vi "Keyence_VS150.vi"(9 "Setting Value":string, 10 "Row No.":string, 11 "Coulumn No.":string) -> (3 "Inspection_Result":bool)   [LabVIEW 2024, in "Keyence_VS150.lvlib"]
doc: "This template is for the Queued Message Handler design pattern.\n\nThe Event Handling Loop generates messages based on user interface actions.\n\nThe Message Handling Loop processes messages generated by the Event Handling Loop, or by other messages. The messages are string values, so new messages can be added easily to the Message Cases case structure in the Message Handling Loop. Each message cluster can also provide an optional value for Message Data, which is a variant that can be converted to whatever message-specific data is required."
uses:
  Keyence_VS150.lvlib
  controls/UI Data.ctl
  Settings/support/Camera.ctl
  <userlib>/_OpenG.lib/array/array.llb/Search 1D Array (String)__ogtk.vi
  <vilib>/Utility/error.llb/Error Cluster From Error Code.vi
  <vilib>/ErrorRing/Error Ring.xnode
  Keysight_34461a/support/Message Queue/Message Queue.lvlib
  support/User Event - Stop/User Event - Stop.lvlib
  support/Message Queue/Message Queue.lvlib
  <userlib>/_OpenG.lib/string/string.llb/openg_string.lvlib
  Launcher/Launcher_DTU.lvlib
  <userlib>/_OpenG.lib/array/array.llb/openg_array.lvlib
  Settings/Setting_Screen.lvlib
panel:
  out "Gray Intensity Value":string
  in  "Row No. 2":string
  in  "Coulumn No. 2":string
  in  "Setting Value 2":string
  in  "Storage 2":string
  in  "Program No 2":string
  out "data 2":string
  out "Get Mode 2":string
  in  "Change_Program":bool
  out "RX/RY":string
  out "RX,RY":string
  out "status":bool
  in  "Trigger":bool
  in  "Total_Result":T1
  out "DTU 2":string[][](array[string])
  out "DTU1":string[][](array[string])
  out "DTU_Failed_Inspections_Array":string[](array[string])
  out "Fail":i32[](array[numeric])
  out "Inspection_names":string[](array[string])
  out "Result_Values":string[](array[string])
  out "DTU_Failed_Inspections":string
  in  "Config":string
  out "queue name 2":string
  out "queue name":string
  in  "ip address":string="169.254.73.187"
  in  "DUT":string
  out "Result Value":string[](array[string])
  out "Array of Strings":string[](array[string])
  out "data out":string
  out "data":string
  out "Get Mode":string
  in  "Program No":string
  in  "Storage":string
  out "Display <Replace Me>":string
  in  "Exit":bool
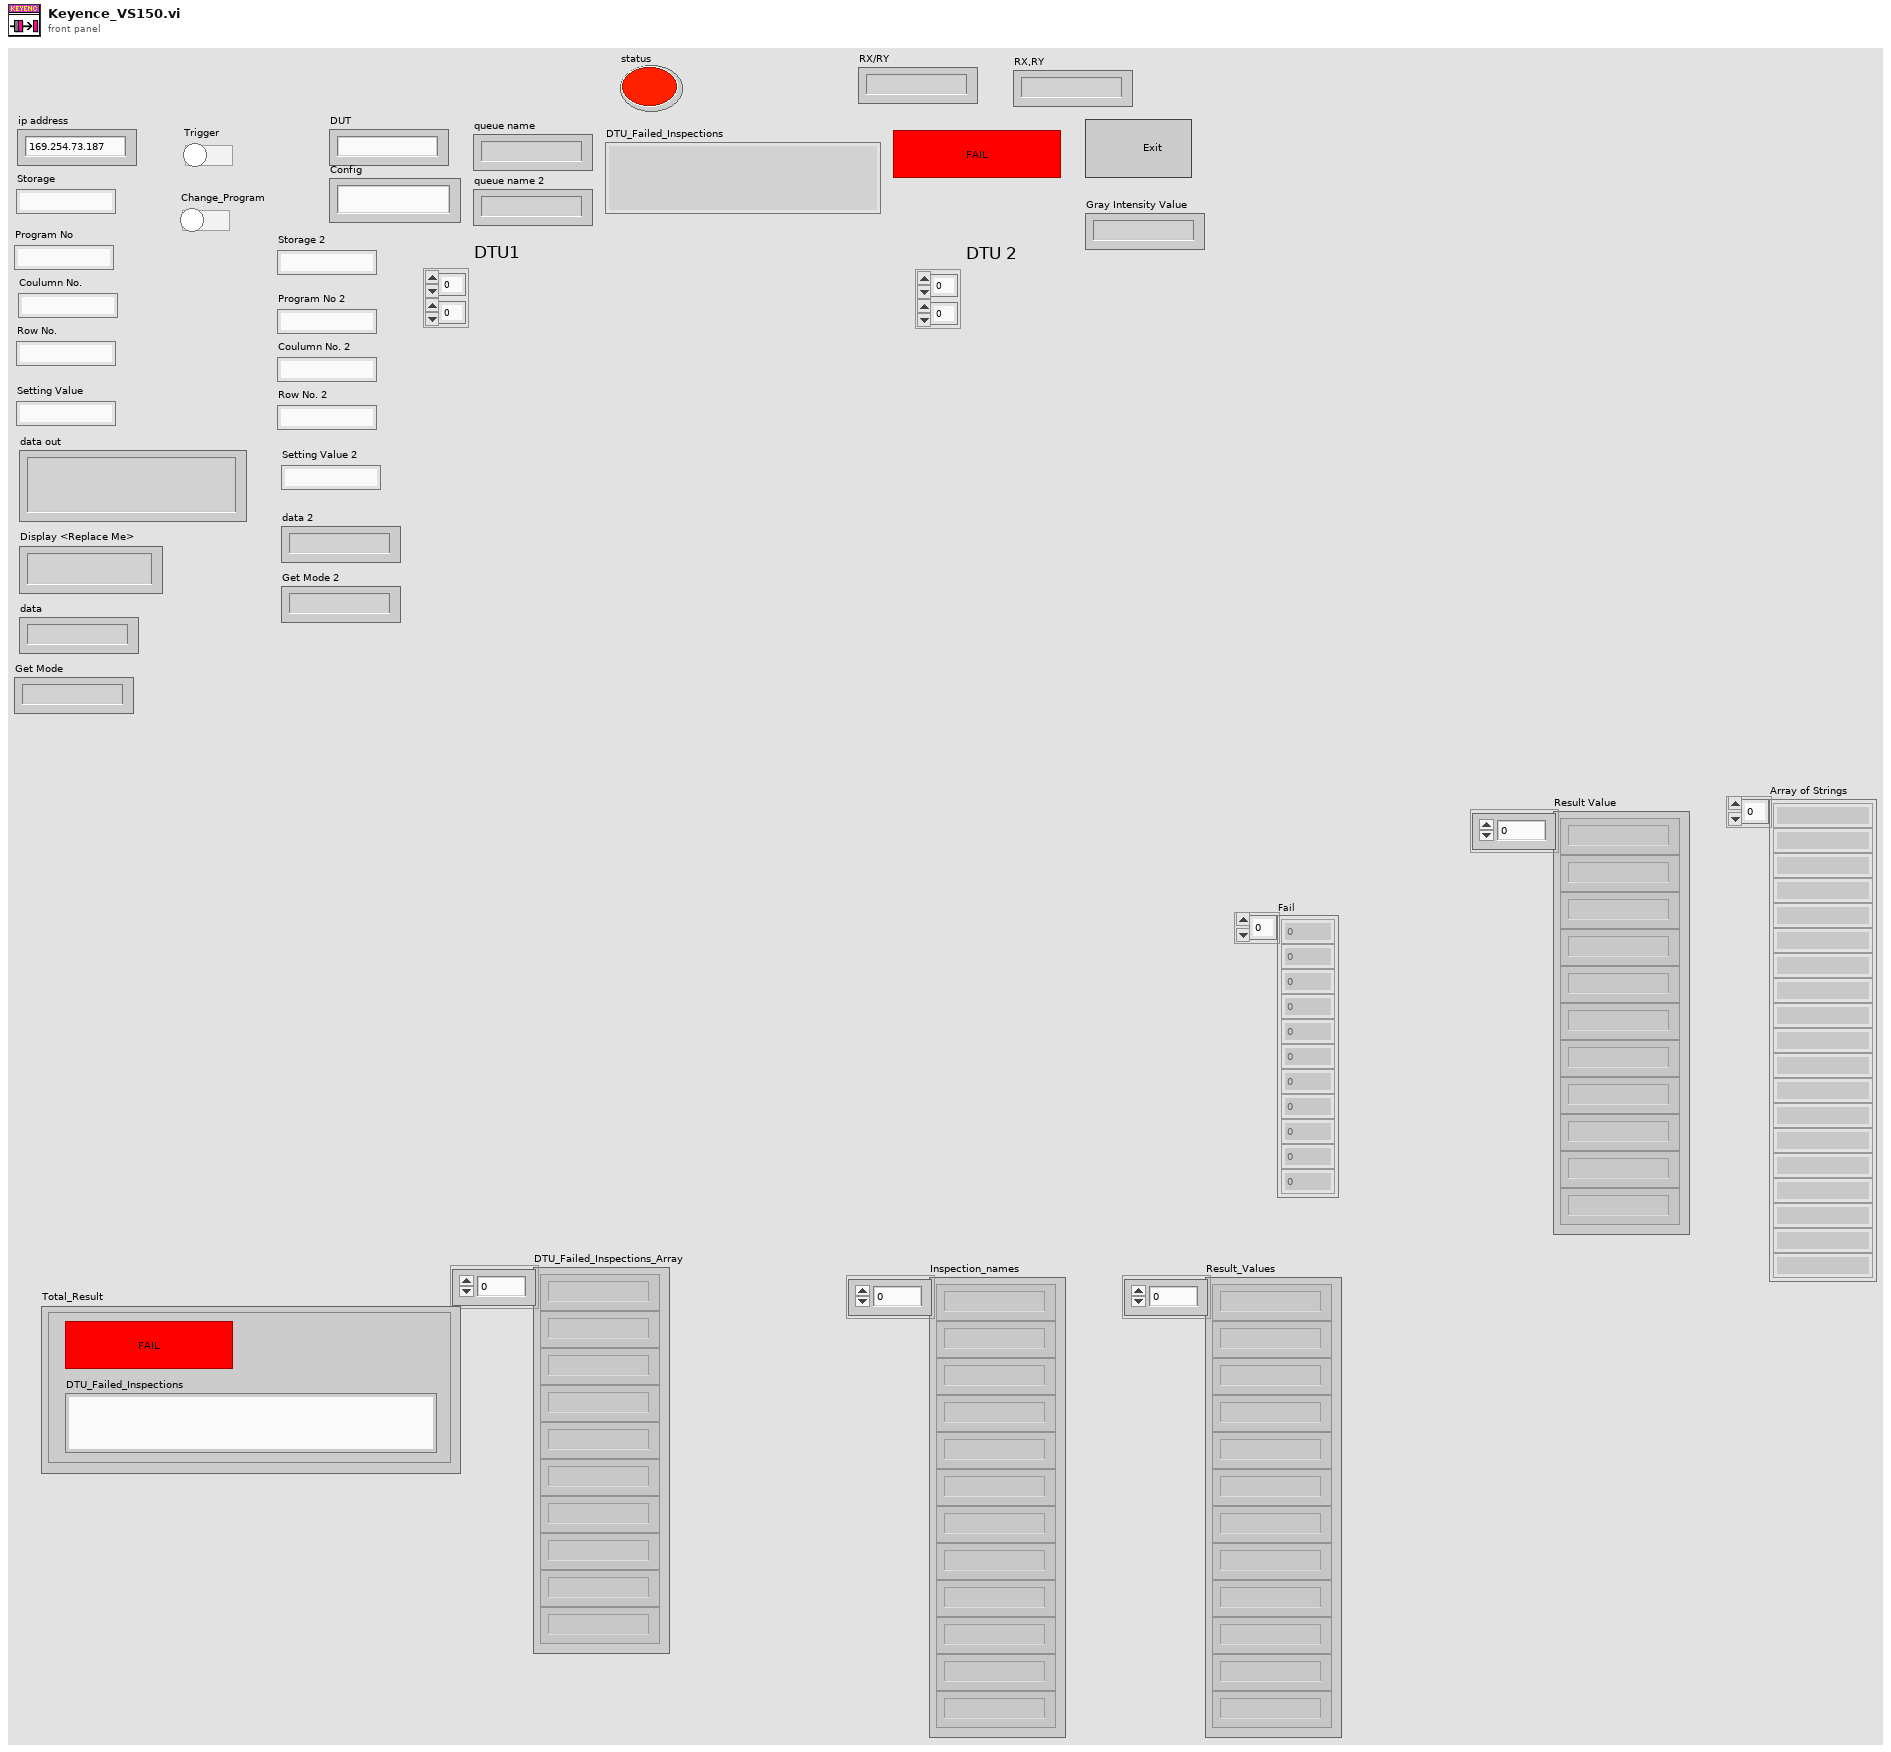
[diagram p1: front panel]
types:
  T1 = cluster{"Inspection_Result 2":bool, "DTU_Failed_Inspections":string}
  T2 = typedef "Keyence_VS150.lvlib/UI Data.ctl" = cluster{"Boolean <Replace Me>":bool, "String <Replace Me>":string, "Numeric <Replace Me>":dbl, "Data Display Ref":refnum<vi>, "Exit Button Ref":refnum<vi>, "connection ID":refnum<k5>, "data out":string, "notifier out":refnum<notifier>, "DUT":string, "Config":string, "Keyence_VS150":refnum<queue>, "Result Value":string[], "Inspection_Result":bool, "Total_Result":cluster{"Inspection_Result 2":bool, "DTU_Failed_Inspections":string}, "Camera":T3, "Camera_Program No":string, "DUT1":string, "DUT2":string}
  T3 = typedef "Setting_Screen.lvlib/Camera.ctl" = cluster{"Trigger":bool, "Prog No.":string, "Delay":bool, "Delay time":dbl, "Storage":string, "Col no.":string, "Row no.":string}
  T4 = typedef "Keyence_VS150.lvlib/Message Queue.lvlib/All Message Queues.ctl" = cluster{"UI":refnum<queue>, "QSM":refnum<queue>}
  T5 = cluster{"Message":string, "Message Data":variant}
  T6 = enum16{"Read", "Write", "All_sections", "All_values", "Remove key&section"}
  T7 = cluster{"Status":string, "Free/inuse":bool, "Action":string}
  T8 = enum16{"Standard", "Buffered", "CRLF", "Immediate"}
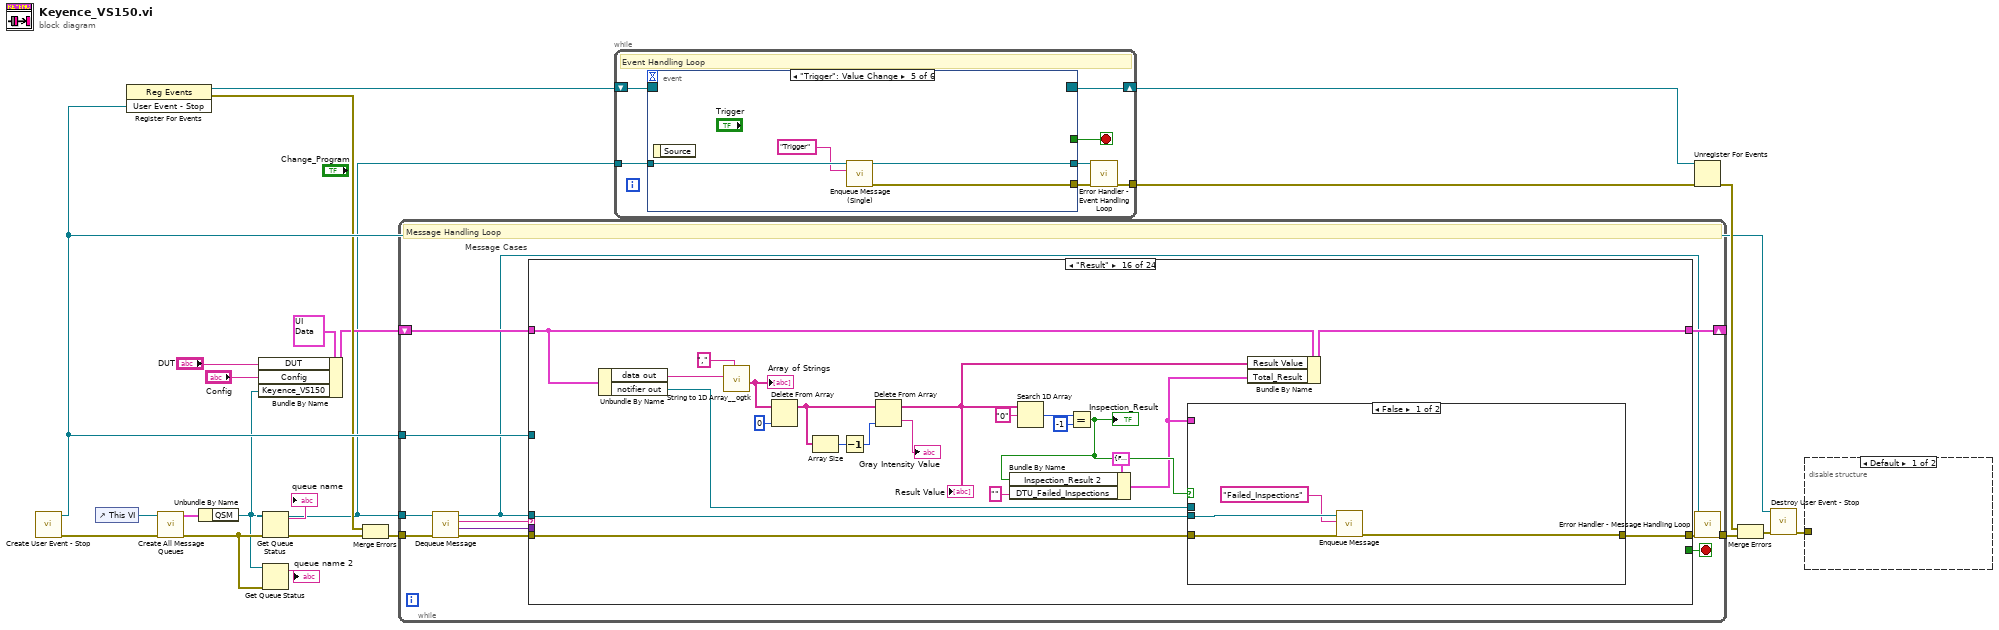
[diagram p0: block diagram]
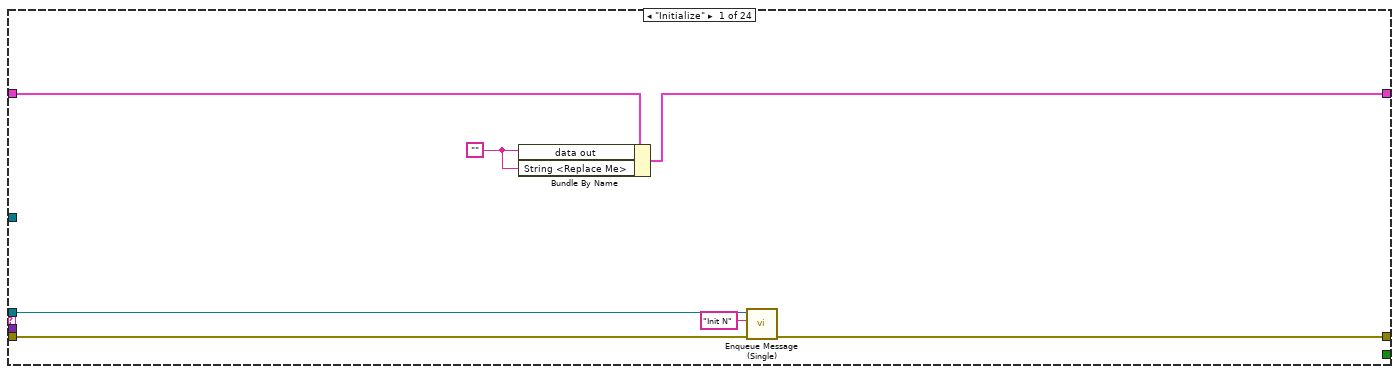
[diagram p2: hidden frame]
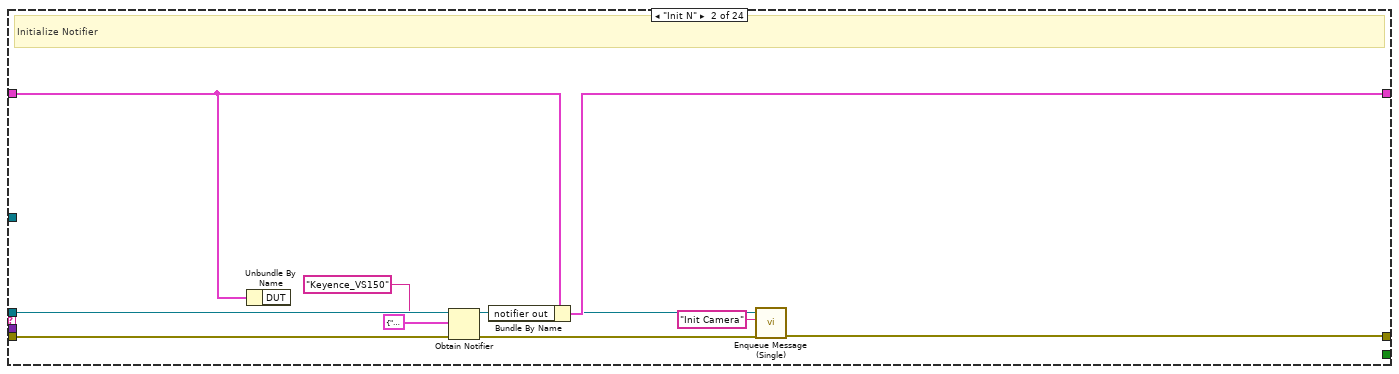
[diagram p3: hidden frame]
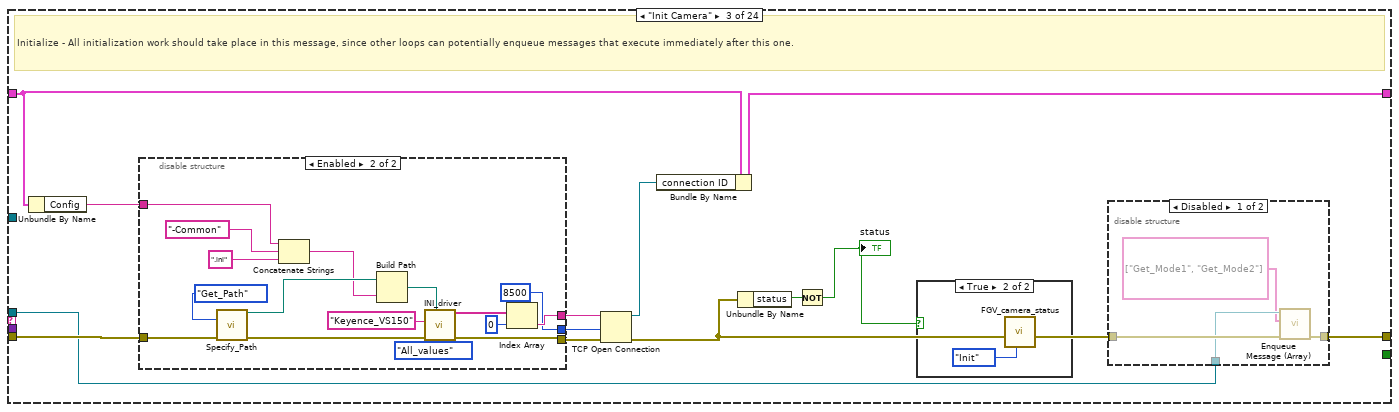
[diagram p4: hidden frame]
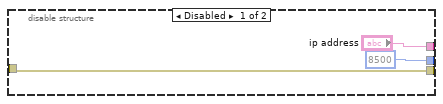
[diagram p7: hidden frame]
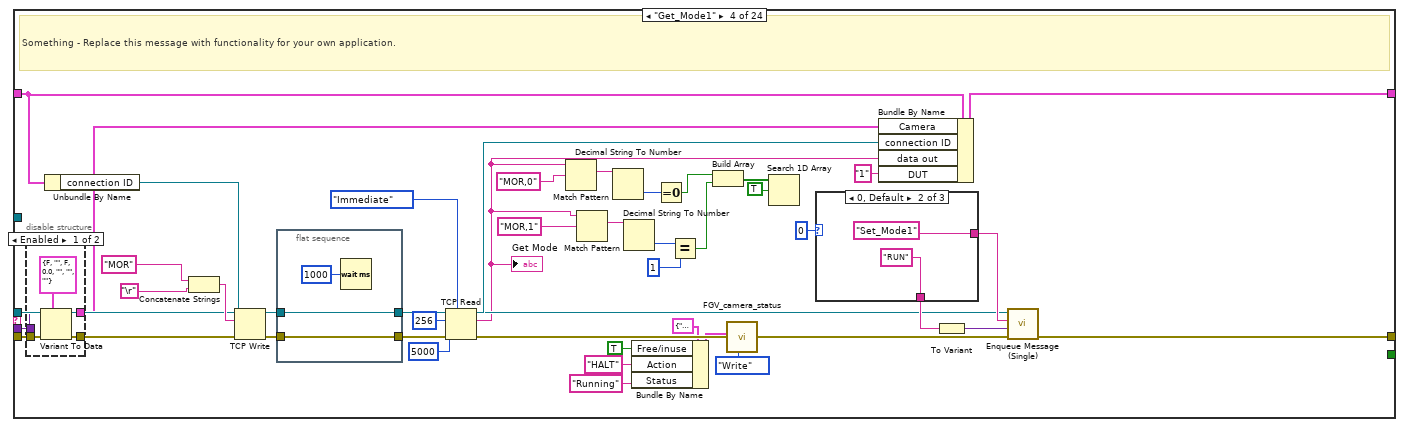
[diagram p8: hidden frame]
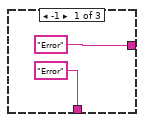
[diagram p10: hidden frame]
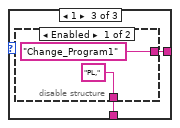
[diagram p11: hidden frame]
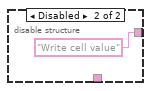
[diagram p12: hidden frame]
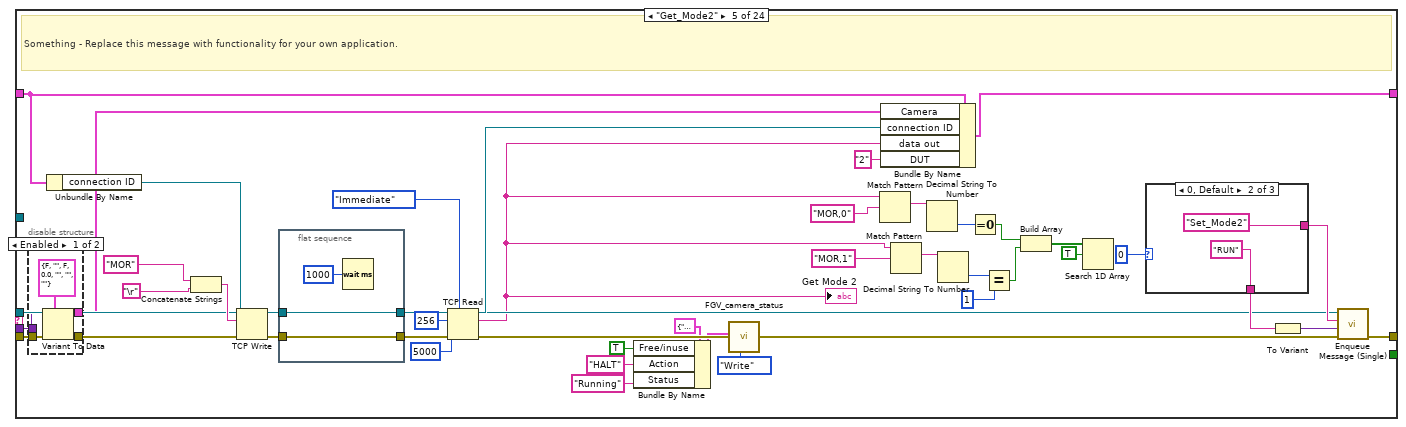
[diagram p13: hidden frame]
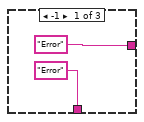
[diagram p15: hidden frame]
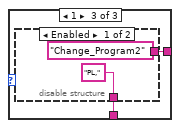
[diagram p16: hidden frame]
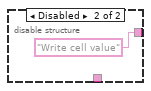
[diagram p17: hidden frame]
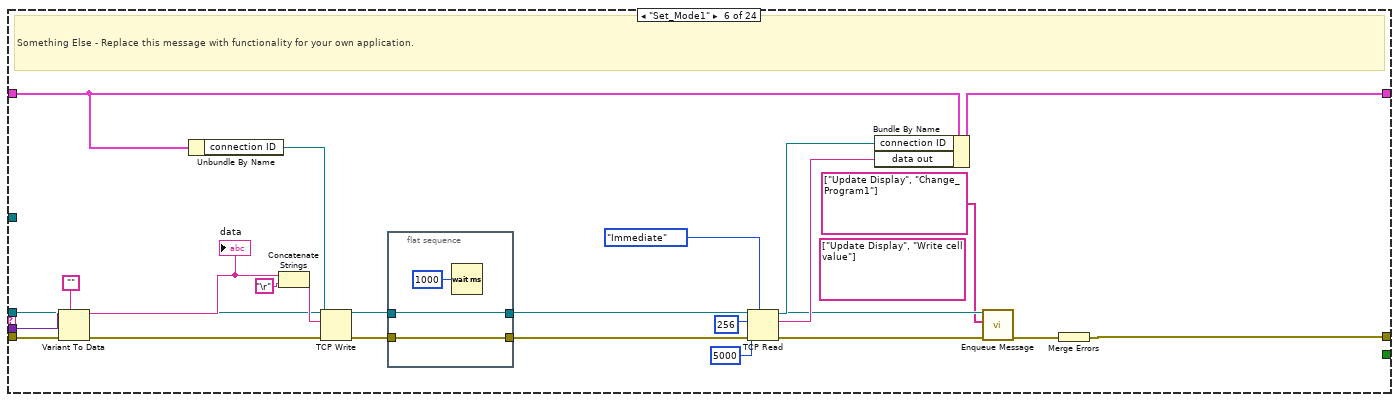
[diagram p18: hidden frame]
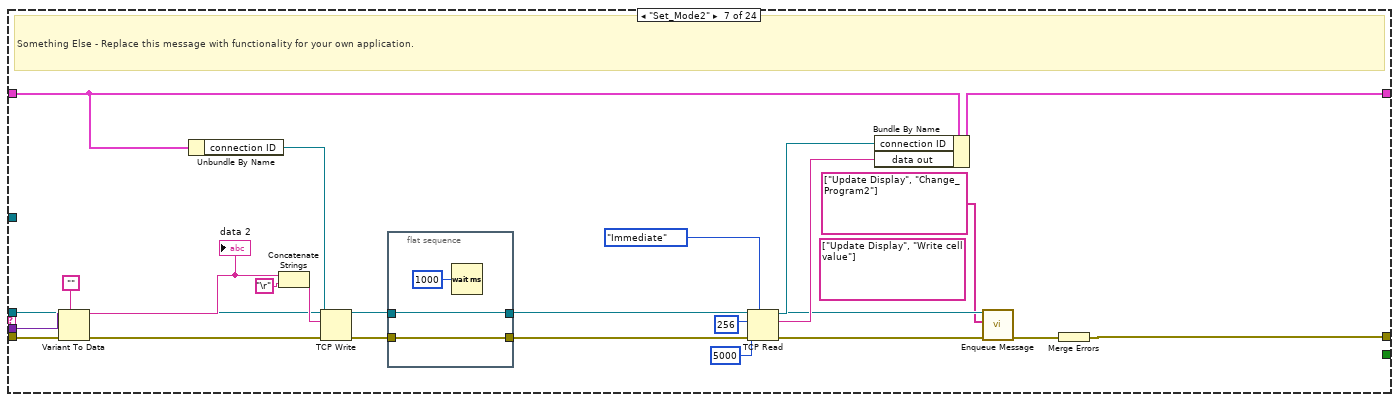
[diagram p19: hidden frame]
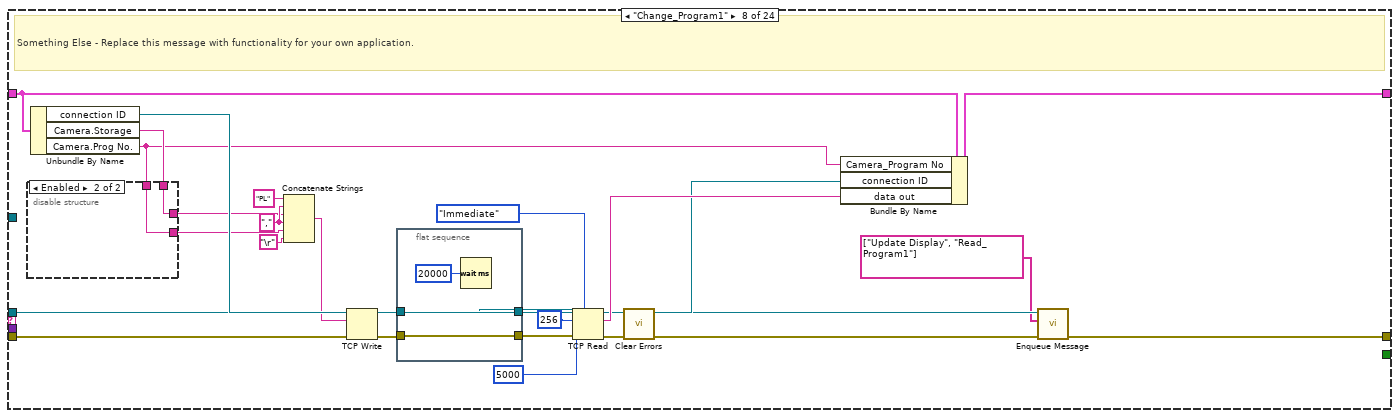
[diagram p20: hidden frame]
diagram:
  n1 = call "Create User Event - Stop.vi"() -> ("error out"=w21:errorcluster, "User Event - Stop"=w14:refnum<user-event>)  [unwired: 10 in]
  n2 = control-ref of="This VI"() -> (w9:refnum<vi>)
  n3 = register-events(w14) -> (reference out=w15:refnum<event-registration>, error out=w12:errorcluster)  [unwired: 2 in]
  n4 = call "Create All Message Queues.vi"("error in (no error)"=w21, "This VI"=w9) -> ("error out"=w3:errorcluster, "Message Queues out"=w23:T4)  [unwired: 8 in]
  n5 = Unbundle By Name(w23) -> ("QSM"=w1:refnum<queue>)
  n6 = Bundle By Name(cluster=T2 {"Boolean <Replace Me>"=FALSE, "String <Replace Me>"="", "Numeric <Replace Me>"=0.0, "Data Display Ref"=refnum, "Exit Button Ref"=refnum, "connection ID"=refnum, "data out"="", "notifier out"=refnum, "DUT"="", "Config"="", "Keyence_VS150"=refnum, "Result Value"=[], "Inspection_Result"=FALSE, "Total_Result"={"Inspection_Result 2"=FALSE, "DTU_Failed_Inspections"=""}, "Camera"={"Trigger"=FALSE, "Prog No."="", "Delay"=FALSE, "Delay time"=0.0, "Storage"="", "Col no."="", "Row no."=""}, "Camera_Program No"="", "DUT1"="", "DUT2"=""} ("Data Cluster"), "DUT"="DUT", "Config"="Config", "Keyence_VS150"=w1) -> (w10:T2)
  n7 = Get Queue Status(queue=w1, error in (no error)=w3) -> (queue out=w5:refnum<queue>, queue name=→"queue name":string, error out=w4:errorcluster)  [unwired: 1 in, 5 out]
  n8 = Get Queue Status(queue=w1, error in (no error)=w3) -> (queue name=→"queue name 2":string)  [unwired: 1 in, 7 out]
  n9 = Merge Errors(w12, w4) -> (w13:errorcluster)
  n10 = while {
    tunnel: w5 -> [w27]
    shift-right: [w34] -> _
    shift-left: w10 -> [w35]
    tunnel: w14 -> [w32]
    tunnel: w13 -> [w31]
    tunnel: [w25] -> w22
    stop <- w33 stop-if-true
    # "Message Handling Loop"
    n11 = call "Dequeue Message.vi"("error in (no error)"=w31, "Message Queue"=w27) -> ("error out"=w30:errorcluster, "Message Data"=w28:variant, "Message"=w29:string, "dup Message Queue"=w26:refnum<queue>)  [unwired: 6 in]
    n12 = case "Message Cases" shown="\"Result\"" w29 {
      selector: w29 -> [_ _ _ _ _ _ _ _ _ _ _ _ _ _ _ _ _ _ _ _ _ _ _ w780]
      tunnel: w26 -> [w37 w45 w54 w115 w176 w218 w245 w283 w316 w337 w384 w451 w502 w546 w574 w604 _ _ _ _ _ w763 w779 _]
      tunnel: w30 -> [w39 w51 w60 w130 w191 w228 w255 w284 w317 w338 w385 w445 w496 w539 w567 w607 w645 w712 w740 w750 w755 w758 w771 _]
      tunnel: [w38 w47 w53 w101 w162 w235 w262 w291 w324 w343 w390 w452 w503 w548 w556 w606 w653 w711 w741 w744 w753 w764 w776 w781] -> w24
      tunnel: w35 -> [w42 w44 w59 w122 w183 w222 w249 w288 w321 w334 w381 w442 w493 w536 w565 w609 w652 w715 w739 w749 w754 w756 w770 w782]
      tunnel: [w40 w49 w64 w121 w182 w221 w248 w287 w320 w340 w387 w441 w492 w535 w564 w608 w652 w715 w739 w749 w754 w756 w770 w782] -> w34
      tunnel: [_ _ _ _ _ _ _ _ _ _ _ _ _ _ _ _ _ _ _ _ _ _ TRUE _] -> w33
      tunnel: w28 -> [_ _ _ w99 w160 w225 w252 _ _ _ _ _ _ _ _ _ _ _ _ w748 _ _ w772 _]
      tunnel: w32 -> [_ _ _ _ _ _ _ _ _ _ _ _ _ _ _ _ _ _ _ _ _ _ w775 _]
      frame "Initialize" {
        w41 = "" ("data out")
        n13 = Bundle By Name(cluster=w42, "data out"=w41, "String <Replace Me>"=w41) -> (w40:T2)
        n14 = call "Enqueue Message (Single).vi"("error in (no error)"=w39, "Message"="Init N", "Message Queue"=w37) -> ("error out"=w38:errorcluster)  [unwired: 7 in, 1 out]
      }
      frame "Init N" {
        # "Initialize Notifier"
        n15 = Unbundle By Name(w44) -> ()  [unwired: 1 out]
        n16 = Obtain Notifier(name (unnamed)="Keyence_VS150", notification data type=T5 {"Message"="", "Message Data"=variant} ("notification"), error in (no error)=w51) -> (notifier out=w50:refnum<notifier>, error out=w48:errorcluster)  [unwired: 1 in, 1 out]
        n17 = Bundle By Name(cluster=w44, "notifier out"=w50) -> (w49:T2)
        n18 = call "Enqueue Message (Single).vi"("error in (no error)"=w48, "Message"="Init Camera", "Message Queue"=w45) -> ("error out"=w47:errorcluster)  [unwired: 7 in, 1 out]
      }
      frame "Init Camera" {
        # "Initialize - All initialization work should take place in this message, since other loops can potentially enqueue messages that execute immediately after this one."
        n19 = Unbundle By Name(w59) -> ("Config"=w58:string)
        n20 = disable-structure shown="Enabled" {
          disable-tunnel: [u16 8500 ("remote port or service name") u16 8500 ("remote port or service name")] -> w65
          disable-tunnel: ["ip address" w76] -> w62
          disable-tunnel: [w71 w77] -> w61
          disable-tunnel: w60 -> [w71 w78]
          disable-tunnel: w58 -> [_ w75]
          frame Disabled {
          }
          frame Enabled {
            n21 = call "Specify_Path.vi"("Path_Enum"=enum16{"Find_Path", "Get_Path"}."Get_Path", "error in (no error)"=w78) -> ("Configurations"=w88:path, "error out"=w85:errorcluster)  [unwired: 6 in, 6 out]
            n22 = Concatenate Strings(w75, "-Common" ("string"), ".ini" ("string")) -> (w80:string)
            n23 = Build Path(base path=w88, name or relative path=w80) -> (appended path=w87:path)
            n24 = call "INI_driver.vi"("Enum"=T6."All_values", "instrument file path"=w87, "error in (no error)"=w85, "Section"="Keyence_VS150") -> ("error out"=w77:errorcluster, "Values out"=w83:string[])  [unwired: 4 in, 2 out]
            n25 = Index Array(array=w83, index=0) -> (element=w76:string)
          }
        }
        n26 = TCP Open Connection(address=w62, remote port or service name=w65, error in (no error)=w61) -> (connection ID=w63:refnum<k5>, error out=w55:errorcluster)  [unwired: 2 in]
        n27 = Bundle By Name(cluster=w59, "connection ID"=w63) -> (w64:T2)
        n28 = Unbundle By Name(w55) -> ("status"=w57:bool)
        n29 = Not(x=w57) -> (.not. x?=w56:bool)
        "status" <- w56
        n30 = case shown="True" w56 {
          frame False {
          }
          frame True {
            n31 = call "FGV_camera_status.vi"("Enum"=enum16{"Init", "Read", "Write"}."Init") -> ()  [unwired: 10 in, 1 out]
          }
        }
        n32 = disable-structure shown="Disabled" {
          disable-tunnel: w55 -> [w69 _]
          disable-tunnel: w54 -> [w68 _]
          disable-tunnel: [w66 _] -> w53
          frame Disabled {
            n33 = call "Enqueue Message (Array).vi"("error in (no error)"=w69, "Message Array"=string[] ["Get_Mode1", "Get_Mode2"], "Message Queue"=w68) -> ("error out"=w66:errorcluster)  [unwired: 7 in, 1 out]
          }
          frame Enabled {
          }
        }
      }
      frame "Get_Mode1" {
        # "Something - Replace this message with functionality for your own application."
        n34 = disable-structure shown="Enabled" {
          disable-tunnel: w130 -> [w138 _]
          disable-tunnel: [w137 _] -> w100
          disable-tunnel: w99 -> [w136 _]
          disable-tunnel: [w134 _] -> w98
          frame Enabled {
            n35 = Variant To Data(error in=w138, type=T3 {"Trigger"=FALSE, "Prog No."="", "Delay"=FALSE, "Delay time"=0.0, "Storage"="", "Col no."="", "Row no."=""} ("Camera"), Variant=w136) -> (data=w134:T3, error out=w137:errorcluster)
          }
          frame Disabled {
          }
        }
        n36 = Unbundle By Name(w122) -> ("connection ID"=w123:refnum<k5>)
        n37 = Concatenate Strings("MOR" ("data in"), "\r") -> (w131:string)
        n38 = TCP Write(connection ID=w123, data in=w131, error in (no error)=w100) -> (connection ID out=w117:refnum<k5>, error out=w114:errorcluster)  [unwired: 1 in, 1 out]
        n39 = flat-sequence {
          tunnel: w117 -> [w141]
          tunnel: [w141] -> w116
          tunnel: w114 -> [w139]
          tunnel: [w139] -> w113
          frame #0 {
            n40 = Wait (ms)(milliseconds to wait=u32 1000) -> ()  [unwired: 1 out]
          }
        }
        n41 = TCP Read(connection ID=w116, bytes to read=256, error in (no error)=w113, 7:T8."Immediate" ("mode (standard)"), 9:5000 ("timeout ms (25000)")) -> (connection ID out=w120:refnum<k5>, data out=w109:string, error out=w126:errorcluster)
        "Get Mode" <- w109
        n42 = Match Pattern(string=w109, regular expression="MOR,0") -> (match substring=w111:string)  [unwired: 1 in, 3 out]
        n43 = Match Pattern(string=w109, regular expression="MOR,1") -> (match substring=w110:string)  [unwired: 1 in, 3 out]
        n44 = Decimal String To Number(string=w111) -> (number=w107:i32)  [unwired: 2 in, 1 out]
        n45 = Decimal String To Number(string=w110) -> (number=w105:i32)  [unwired: 2 in, 1 out]
        n46 = Bundle By Name(cluster=T7 {"Status"="", "Free/inuse"=FALSE, "Action"=""} ("Write"), "Free/inuse"=TRUE, "Action"="HALT", "Status"="Running") -> (w94:T7)
        n47 = Equal To 0?(x=w107) -> (x = 0?=w106:bool)
        n48 = Equal?(x=w105, y=1) -> (x = y?=w103:bool)
        n49 = Build Array(w106, w103) -> (w125:bool[])
        n50 = call "FGV_camera_status.vi"("Enum"=enum16{"Init", "Read", "Write"}."Write", "Write"=w94) -> ()  [unwired: 9 in, 1 out]
        n51 = Search 1D Array(1D array=w125, element=TRUE) -> ()  [unwired: 1 in, 1 out]
        n52 = case shown="0, Default" 0 ("index of element") {
          tunnel: ["Error" "Set_Mode1" w147] -> w124
          tunnel: ["Error" "RUN" w146] -> w119
          frame -1 {
          }
          frame 0, Default {
          }
          frame 1 {
            n53 = disable-structure shown="Enabled" {
              disable-tunnel: ["Change_Program1" "Write cell value"] -> w147
              disable-tunnel: ["PL," _] -> w146
              frame Enabled {
              }
              frame Disabled {
              }
            }
          }
        }
        n54 = Bundle By Name(cluster=w122, "Camera"=w98, "connection ID"=w120, "data out"=w109, "DUT"="1" ("DUT1")) -> (w121:T2)
        n55 = To Variant(anything=w119) -> (Variant=w118:variant)
        n56 = call "Enqueue Message (Single).vi"("error in (no error)"=w126, "Message Data"=w118, "Message"=w124, "Message Queue"=w115) -> ("error out"=w101:errorcluster)  [unwired: 6 in, 1 out]
      }
      frame "Get_Mode2" {
        # "Something - Replace this message with functionality for your own application."
        n57 = disable-structure shown="Enabled" {
          disable-tunnel: w191 -> [w199 _]
          disable-tunnel: [w198 _] -> w161
          disable-tunnel: w160 -> [w197 _]
          disable-tunnel: [w196 _] -> w159
          frame Enabled {
            n58 = Variant To Data(error in=w199, type=T3 {"Trigger"=FALSE, "Prog No."="", "Delay"=FALSE, "Delay time"=0.0, "Storage"="", "Col no."="", "Row no."=""} ("Camera"), Variant=w197) -> (data=w196:T3, error out=w198:errorcluster)
          }
          frame Disabled {
          }
        }
        n59 = Unbundle By Name(w183) -> ("connection ID"=w184:refnum<k5>)
        n60 = Concatenate Strings("MOR" ("data in"), "\r") -> (w192:string)
        n61 = TCP Write(connection ID=w184, data in=w192, error in (no error)=w161) -> (connection ID out=w178:refnum<k5>, error out=w175:errorcluster)  [unwired: 1 in, 1 out]
        n62 = flat-sequence {
          tunnel: w178 -> [w202]
          tunnel: [w202] -> w177
          tunnel: w175 -> [w200]
          tunnel: [w200] -> w174
          frame #0 {
            n63 = Wait (ms)(milliseconds to wait=u32 1000) -> ()  [unwired: 1 out]
          }
        }
        n64 = TCP Read(connection ID=w177, bytes to read=256, error in (no error)=w174, 7:T8."Immediate" ("mode (standard)"), 9:5000 ("timeout ms (25000)")) -> (connection ID out=w181:refnum<k5>, data out=w170:string, error out=w187:errorcluster)
        "Get Mode 2" <- w170
        n65 = Bundle By Name(cluster=T7 {"Status"="", "Free/inuse"=FALSE, "Action"=""} ("Write"), "Free/inuse"=TRUE, "Action"="HALT", "Status"="Running") -> (w155:T7)
        n66 = call "FGV_camera_status.vi"("Enum"=enum16{"Init", "Read", "Write"}."Write", "Write"=w155) -> ()  [unwired: 9 in, 1 out]
        n67 = Match Pattern(string=w170, regular expression="MOR,0") -> (match substring=w172:string)  [unwired: 1 in, 3 out]
        n68 = Bundle By Name(cluster=w183, "Camera"=w159, "connection ID"=w181, "data out"=w170, "DUT"="2" ("DUT1")) -> (w182:T2)
        n69 = Match Pattern(string=w170, regular expression="MOR,1") -> (match substring=w171:string)  [unwired: 1 in, 3 out]
        n70 = Decimal String To Number(string=w172) -> (number=w168:i32)  [unwired: 2 in, 1 out]
        n71 = Decimal String To Number(string=w171) -> (number=w166:i32)  [unwired: 2 in, 1 out]
        n72 = Equal To 0?(x=w168) -> (x = 0?=w167:bool)
        n73 = Equal?(x=w166, y=1) -> (x = y?=w164:bool)
        n74 = Build Array(w167, w164) -> (w186:bool[])
        n75 = Search 1D Array(1D array=w186, element=TRUE) -> ()  [unwired: 1 in, 1 out]
        n76 = case shown="0, Default" 0 ("index of element") {
          tunnel: ["Error" "Set_Mode2" w208] -> w185
          tunnel: ["Error" "RUN" w207] -> w180
          frame -1 {
          }
          frame 0, Default {
          }
          frame 1 {
            n77 = disable-structure shown="Enabled" {
              disable-tunnel: ["Change_Program2" "Write cell value"] -> w208
              disable-tunnel: ["PL," _] -> w207
              frame Enabled {
              }
              frame Disabled {
              }
            }
          }
        }
        n78 = To Variant(anything=w180) -> (Variant=w179:variant)
        n79 = call "Enqueue Message (Single).vi"("error in (no error)"=w187, "Message Data"=w179, "Message"=w185, "Message Queue"=w176) -> ("error out"=w162:errorcluster)  [unwired: 6 in, 1 out]
      }
      frame "Set_Mode1" {
        (unwired) string[] ["Update Display", "Write cell value"]
        # "Something Else - Replace this message with functionality for your own application."
        n80 = Variant To Data(error in=w228, type="", Variant=w225) -> (data=w224:string, error out=w227:errorcluster)
        "data" <- w224
        n81 = Unbundle By Name(w222) -> ("connection ID"=w213:refnum<k5>)
        n82 = Concatenate Strings(w224, "\r") -> (w232:string)
        n83 = TCP Write(connection ID=w213, data in=w232, error in (no error)=w227) -> (connection ID out=w215:refnum<k5>, error out=w217:errorcluster)  [unwired: 1 in, 1 out]
        n84 = flat-sequence {
          tunnel: w217 -> [w237]
          tunnel: [w237] -> w216
          tunnel: w215 -> [w236]
          tunnel: [w236] -> w214
          frame #0 {
            n85 = Wait (ms)(milliseconds to wait=u32 1000) -> ()  [unwired: 1 out]
          }
        }
        n86 = TCP Read(connection ID=w214, bytes to read=256, error in (no error)=w216, 7:T8."Immediate" ("mode (standard)"), 9:5000 ("timeout ms (25000)")) -> (connection ID out=w220:refnum<k5>, data out=w219:string, error out=w223:errorcluster)
        n87 = Bundle By Name(cluster=w222, "connection ID"=w220, "data out"=w219) -> (w221:T2)
        n88 = call-poly "Enqueue Message.vi"("error in (no error)"=w223, "Message Array"=string[] ["Update Display", "Change_Program1"], "Message Queue"=w218) -> ("error out"=w234:errorcluster)  [unwired: 7 in, 1 out]
        n89 = Merge Errors(w234) -> (w235:errorcluster)
      }
      frame "Set_Mode2" {
        (unwired) string[] ["Update Display", "Write cell value"]
        # "Something Else - Replace this message with functionality for your own application."
        n90 = Variant To Data(error in=w255, type="", Variant=w252) -> (data=w251:string, error out=w254:errorcluster)
        "data 2" <- w251
        n91 = Unbundle By Name(w249) -> ("connection ID"=w240:refnum<k5>)
        n92 = Concatenate Strings(w251, "\r") -> (w259:string)
        n93 = TCP Write(connection ID=w240, data in=w259, error in (no error)=w254) -> (connection ID out=w242:refnum<k5>, error out=w244:errorcluster)  [unwired: 1 in, 1 out]
        n94 = flat-sequence {
          tunnel: w244 -> [w264]
          tunnel: [w264] -> w243
          tunnel: w242 -> [w263]
          tunnel: [w263] -> w241
          frame #0 {
            n95 = Wait (ms)(milliseconds to wait=u32 1000) -> ()  [unwired: 1 out]
          }
        }
        n96 = TCP Read(connection ID=w241, bytes to read=256, error in (no error)=w243, 7:T8."Immediate" ("mode (standard)"), 9:5000 ("timeout ms (25000)")) -> (connection ID out=w247:refnum<k5>, data out=w246:string, error out=w250:errorcluster)
        n97 = Bundle By Name(cluster=w249, "connection ID"=w247, "data out"=w246) -> (w248:T2)
        n98 = call-poly "Enqueue Message.vi"("error in (no error)"=w250, "Message Array"=string[] ["Update Display", "Change_Program2"], "Message Queue"=w245) -> ("error out"=w261:errorcluster)  [unwired: 7 in, 1 out]
        n99 = Merge Errors(w261) -> (w262:errorcluster)
      }
      frame "Change_Program1" {
        w270 = "," ("string")
        # "Something Else - Replace this message with functionality for your own application."
        n100 = Unbundle By Name(w288) -> ("connection ID"=w290:refnum<k5>, "Camera.Storage"=w267:string, "Camera.Prog No."=w266:string)
        n101 = disable-structure shown="Enabled" {
          disable-tunnel: ["Storage" w295] -> w269
          disable-tunnel: ["Program No" w294] -> w268
          disable-tunnel: w267 -> [_ w295]
          disable-tunnel: w266 -> [_ w294]
          frame Disabled {
          }
          frame Enabled {
          }
        }
        n102 = Concatenate Strings("PL" ("string"), w270, w269, w270, w268, "\r") -> (w281:string)
        n103 = TCP Write(connection ID=w290, data in=w281, error in (no error)=w284) -> (connection ID out=w275:refnum<k5>, error out=w274:errorcluster)  [unwired: 1 in, 1 out]
        n104 = flat-sequence {
          tunnel: w275 -> [w298]
          tunnel: [w298] -> w272
          tunnel: w274 -> [w296]
          tunnel: [w296] -> w273
          frame #0 {
            n105 = Wait (ms)(milliseconds to wait=u32 20000) -> ()  [unwired: 1 out]
          }
        }
        n106 = TCP Read(connection ID=w272, bytes to read=256, error in (no error)=w273, 7:T8."Immediate" ("mode (standard)"), 9:5000 ("timeout ms (25000)")) -> (connection ID out=w285:refnum<k5>, data out=w286:string, error out=w276:errorcluster)
        n107 = call <vilib>:"Clear Errors.vi"("error in (no error)"=w276) -> ("error out"=w289:errorcluster)  [unwired: 5 in, 1 out]
        n108 = Bundle By Name(cluster=w288, "Camera_Program No"=w266, "connection ID"=w285, "data out"=w286) -> (w287:T2)
        n109 = call-poly "Enqueue Message.vi"("error in (no error)"=w289, "Message Array"=string[] ["Update Display", "Read_Program1"], "Message Queue"=w283) -> ("error out"=w291:errorcluster)  [unwired: 7 in, 1 out]
      }
      frame "Change_Program2" {
        w303 = "," ("string")
        # "Something Else - Replace this message with functionality for your own application."
        n110 = Unbundle By Name(w321) -> ("connection ID"=w323:refnum<k5>, "Camera.Storage"=w300:string, "Camera.Prog No."=w299:string)
        n111 = disable-structure shown="Enabled" {
          disable-tunnel: ["Storage 2" w328] -> w302
          disable-tunnel: ["Program No 2" w327] -> w301
          disable-tunnel: w300 -> [_ w328]
          disable-tunnel: w299 -> [_ w327]
          frame Disabled {
          }
          frame Enabled {
          }
        }
        n112 = Concatenate Strings("PL" ("string"), w303, w302, w303, w301, "\r") -> (w314:string)
        n113 = TCP Write(connection ID=w323, data in=w314, error in (no error)=w317) -> (connection ID out=w308:refnum<k5>, error out=w307:errorcluster)  [unwired: 1 in, 1 out]
        n114 = flat-sequence {
          tunnel: w308 -> [w331]
          tunnel: [w331] -> w305
          tunnel: w307 -> [w329]
          tunnel: [w329] -> w306
          frame #0 {
            n115 = Wait (ms)(milliseconds to wait=u32 20000) -> ()  [unwired: 1 out]
          }
        }
        n116 = TCP Read(connection ID=w305, bytes to read=256, error in (no error)=w306, 7:T8."Immediate" ("mode (standard)"), 9:5000 ("timeout ms (25000)")) -> (connection ID out=w318:refnum<k5>, data out=w319:string, error out=w309:errorcluster)
        n117 = call <vilib>:"Clear Errors.vi"("error in (no error)"=w309) -> ("error out"=w322:errorcluster)  [unwired: 5 in, 1 out]
        n118 = Bundle By Name(cluster=w321, "Camera_Program No"=w299, "connection ID"=w318, "data out"=w319) -> (w320:T2)
        n119 = call-poly "Enqueue Message.vi"("error in (no error)"=w322, "Message Array"=string[] ["Update Display", "Read_Program2"], "Message Queue"=w316) -> ("error out"=w324:errorcluster)  [unwired: 7 in, 1 out]
      }
      frame "Read_Program1" {
        # "Something Else - Replace this message with functionality for your own application."
        n120 = Unbundle By Name(w334) -> ("connection ID"=w342:refnum<k5>)
        n121 = Unbundle By Name(w334) -> ("Camera_Program No"=w333:string)
        n122 = for {
          N: 3 -> [_]
          tunnel: [w357] -> w335
          shift-right: [w366] -> w339
          shift-left: w342 -> [w368]
          shift-right: [w356] -> w341
          shift-left: w338 -> [w365]
          tunnel: w333 -> [w352]
          tunnel: [w355] -> w332
          stop <- w355 stop-if-true
          n123 = Concatenate Strings("PR" ("string"), "\r") -> (w373:string)
          n124 = TCP Write(connection ID=w368, data in=w373, error in (no error)=w365) -> (connection ID out=w364:refnum<k5>, error out=w363:errorcluster)  [unwired: 1 in, 1 out]
          n125 = flat-sequence {
            tunnel: w364 -> [w378]
            tunnel: [w378] -> w361
            tunnel: w363 -> [w376]
            tunnel: [w376] -> w362
            frame #0 {
              n126 = Wait (ms)(milliseconds to wait=u32 1000) -> ()  [unwired: 1 out]
            }
          }
          n127 = disable-structure shown="Enabled" {
            disable-tunnel: [w374 w375] -> w353
            disable-tunnel: w352 -> [_ w375]
            frame Disabled {
              n128 = local read "Program No"() -> (w374:string)
            }
            frame Enabled {
            }
          }
          n129 = TCP Read(connection ID=w361, bytes to read=256, error in (no error)=w362, 7:T8."Immediate" ("mode (standard)"), 9:5000 ("timeout ms (25000)")) -> (connection ID out=w366:refnum<k5>, data out=w357:string, error out=w367:errorcluster)
          n130 = String Subset(string=w357, offset (0)=5, length (rest)=1 ("length (rest)")) -> (substring=w359:string)
          n131 = call <vilib>:"Clear Errors.vi"("error in (no error)"=w367) -> ("error out"=w356:errorcluster)  [unwired: 5 in, 1 out]
          n132 = Equal?(x=w353, y=w359) -> (x = y?=w355:bool)
        }
        n133 = case shown="True" w332 {
          tunnel: [w346 w351] -> w343
          tunnel: w341 -> [w347 w350]
          tunnel: w337 -> [w345 w349]
          frame False {
            n134 = call-poly "Enqueue Message.vi"("error in (no error)"=w347, "Message"="Change_Program1", "Message Queue"=w345) -> ("error out"=w346:errorcluster)  [unwired: 7 in, 1 out]
          }
          frame True {
            n135 = call-poly "Enqueue Message.vi"("error in (no error)"=w350, "Message Array"=string[] ["Update Display", "Write cell value1"], "Message Queue"=w349) -> ("error out"=w351:errorcluster)  [unwired: 7 in, 1 out]
          }
        }
        n136 = Bundle By Name(cluster=w334, "connection ID"=w339, "data out"=w335) -> (w340:T2)
      }
      frame "Read_Program2" {
        # "Something Else - Replace this message with functionality for your own application."
        n137 = Unbundle By Name(w381) -> ("connection ID"=w389:refnum<k5>)
        n138 = Unbundle By Name(w381) -> ("Camera_Program No"=w379:string)
        n139 = for {
          N: 3 -> [_]
          tunnel: [w404] -> w382
          shift-right: [w413] -> w386
          shift-left: w389 -> [w415]
          shift-right: [w403] -> w388
          shift-left: w385 -> [w412]
          tunnel: [w402] -> w380
          tunnel: w379 -> [w400]
          stop <- w402 stop-if-true
          n140 = Concatenate Strings("PR" ("string"), "\r") -> (w420:string)
          n141 = TCP Write(connection ID=w415, data in=w420, error in (no error)=w412) -> (connection ID out=w411:refnum<k5>, error out=w410:errorcluster)  [unwired: 1 in, 1 out]
          n142 = flat-sequence {
            tunnel: w411 -> [w425]
            tunnel: [w425] -> w408
            tunnel: w410 -> [w423]
            tunnel: [w423] -> w409
            frame #0 {
              n143 = Wait (ms)(milliseconds to wait=u32 1000) -> ()  [unwired: 1 out]
            }
          }
          n144 = disable-structure shown="Enabled" {
            disable-tunnel: [w421 w422] -> w399
            disable-tunnel: w400 -> [_ w422]
            frame Disabled {
              n145 = local read "Program No"() -> (w421:string)
            }
            frame Enabled {
            }
          }
          n146 = TCP Read(connection ID=w408, bytes to read=256, error in (no error)=w409, 7:T8."Immediate" ("mode (standard)"), 9:5000 ("timeout ms (25000)")) -> (connection ID out=w413:refnum<k5>, data out=w404:string, error out=w414:errorcluster)
          n147 = String Subset(string=w404, offset (0)=5, length (rest)=1 ("length (rest)")) -> (substring=w406:string)
          n148 = call <vilib>:"Clear Errors.vi"("error in (no error)"=w414) -> ("error out"=w403:errorcluster)  [unwired: 5 in, 1 out]
          n149 = Equal?(x=w399, y=w406) -> (x = y?=w402:bool)
        }
        n150 = case shown="True" w380 {
          tunnel: [w393 w398] -> w390
          tunnel: w388 -> [w394 w397]
          tunnel: w384 -> [w392 w396]
          frame False {
            n151 = call-poly "Enqueue Message.vi"("error in (no error)"=w394, "Message"="Change_Program2", "Message Queue"=w392) -> ("error out"=w393:errorcluster)  [unwired: 7 in, 1 out]
          }
          frame True {
            n152 = call-poly "Enqueue Message.vi"("error in (no error)"=w397, "Message Array"=string[] ["Update Display", "Write cell value2"], "Message Queue"=w396) -> ("error out"=w398:errorcluster)  [unwired: 7 in, 1 out]
          }
        }
        n153 = Bundle By Name(cluster=w381, "connection ID"=w386, "data out"=w382) -> (w387:T2)
      }
      frame "Write cell value1" {
        w438 = "," ("string")
        # "Something Else - Replace this message with functionality for your own application."
        n154 = Unbundle By Name(w442) -> ("notifier out"=w431:refnum<notifier>, "connection ID"=w443:refnum<k5>, "DUT"=w432:string, "Camera.Col no."=w429:string, "Camera.Row no."=w427:string)
        n155 = disable-structure shown="Enabled" {
          disable-tunnel: w429 -> [_ w456]
          disable-tunnel: ["Coulumn No." w456] -> w428
          disable-tunnel: w427 -> [_ w455]
          disable-tunnel: ["Row No." w455] -> w426
          frame Disabled {
          }
          frame Enabled {
          }
        }
        n156 = disable-structure shown="Enabled" {
          disable-tunnel: [w472 "Setting Value"] -> w433
          disable-tunnel: w432 -> [w472 _]
          frame Enabled {
          }
          frame Disabled {
          }
        }
        n157 = Concatenate Strings("CWN," ("data in"), w428, w438, w426, w438, w433, "\r") -> (w450:string)
        n158 = TCP Write(connection ID=w443, data in=w450, error in (no error)=w445) -> (connection ID out=w437:refnum<k5>, error out=w436:errorcluster)  [unwired: 1 in, 1 out]
        n159 = flat-sequence {
          tunnel: w437 -> [w476]
          tunnel: [w476] -> w434
          tunnel: w436 -> [w474]
          tunnel: [w474] -> w435
          frame #0 {
            n160 = Wait (ms)(milliseconds to wait=u32 1000) -> ()  [unwired: 1 out]
          }
        }
        n161 = TCP Read(connection ID=w434, bytes to read=256, error in (no error)=w435, 7:T8."Immediate" ("mode (standard)"), 9:5000 ("timeout ms (25000)")) -> (connection ID out=w439:refnum<k5>, data out=w440:string, error out=w444:errorcluster)
        n162 = disable-structure shown="Enabled" {
          disable-tunnel: [w461 w464] -> w452
          disable-tunnel: w451 -> [w459 _]
          disable-tunnel: w444 -> [w458 w463]
          disable-tunnel: w431 -> [_ w462]
          frame Disabled {
            n163 = call-poly "Enqueue Message.vi"("error in (no error)"=w458, "Message Array"=string[] ["Update Display", "Trigger"], "Message Queue"=w459) -> ("error out"=w460:errorcluster)  [unwired: 7 in, 1 out]
            n164 = Merge Errors(w460) -> (w461:errorcluster)
          }
          frame Enabled {
            n165 = Unbundle By Name(w463) -> ("status"=w471:bool)
            n166 = Select(t="Error" ("f"), s=w471, f="Step_Done" ("Message")) -> (s? t:f=w467:string)
            n167 = Bundle By Name(cluster=T5 {"Message"="", "Message Data"=variant} ("notification"), "Message"=w467) -> (w466:T5)
            n168 = call <vilib>:"Clear Errors.vi"("error in (no error)"=w463) -> ("error out"=w465:errorcluster)  [unwired: 5 in, 1 out]
            n169 = Send Notification(notification=w466, notifier=w462, error in (no error)=w465) -> (error out=w464:errorcluster)  [unwired: 1 out]
          }
        }
        n170 = Bundle By Name(cluster=w442, "connection ID"=w439, "data out"=w440) -> (w441:T2)
      }
      frame "Write cell value2" {
        w488 = "," ("string")
        # "Something Else - Replace this message with functionality for your own application."
        n171 = Unbundle By Name(w493) -> ("notifier out"=w481:refnum<notifier>, "connection ID"=w494:refnum<k5>, "DUT"=w482:string, "Camera.Col no."=w478:string, "Camera.Row no."=w477:string)
        n172 = disable-structure shown="Enabled" {
          disable-tunnel: ["Coulumn No. 2" w507] -> w480
          disable-tunnel: ["Row No. 2" w506] -> w479
          disable-tunnel: w478 -> [_ w507]
          disable-tunnel: w477 -> [_ w506]
          frame Disabled {
          }
          frame Enabled {
          }
        }
        n173 = disable-structure shown="Enabled" {
          disable-tunnel: [w523 "Setting Value 2"] -> w483
          disable-tunnel: w482 -> [w523 _]
          frame Enabled {
          }
          frame Disabled {
          }
        }
        n174 = Concatenate Strings("CWN," ("data in"), w480, w488, w479, w488, w483, "\r") -> (w501:string)
        n175 = TCP Write(connection ID=w494, data in=w501, error in (no error)=w496) -> (connection ID out=w487:refnum<k5>, error out=w486:errorcluster)  [unwired: 1 in, 1 out]
        n176 = flat-sequence {
          tunnel: w487 -> [w527]
          tunnel: [w527] -> w484
          tunnel: w486 -> [w525]
          tunnel: [w525] -> w485
          frame #0 {
            n177 = Wait (ms)(milliseconds to wait=u32 1000) -> ()  [unwired: 1 out]
          }
        }
        n178 = TCP Read(connection ID=w484, bytes to read=256, error in (no error)=w485, 7:T8."Immediate" ("mode (standard)"), 9:5000 ("timeout ms (25000)")) -> (connection ID out=w490:refnum<k5>, data out=w491:string, error out=w495:errorcluster)
        n179 = disable-structure shown="Enabled" {
          disable-tunnel: [w512 w515] -> w503
          disable-tunnel: w502 -> [w510 _]
          disable-tunnel: w495 -> [w509 w514]
          disable-tunnel: w481 -> [_ w513]
          frame Disabled {
            n180 = call-poly "Enqueue Message.vi"("error in (no error)"=w509, "Message Array"=string[] ["Update Display", "Trigger"], "Message Queue"=w510) -> ("error out"=w511:errorcluster)  [unwired: 7 in, 1 out]
            n181 = Merge Errors(w511) -> (w512:errorcluster)
          }
          frame Enabled {
            n182 = Unbundle By Name(w514) -> ("status"=w522:bool)
            n183 = Select(t="Error" ("f"), s=w522, f="Step_Done" ("Message")) -> (s? t:f=w518:string)
            n184 = Bundle By Name(cluster=T5 {"Message"="", "Message Data"=variant} ("notification"), "Message"=w518) -> (w517:T5)
            n185 = call <vilib>:"Clear Errors.vi"("error in (no error)"=w514) -> ("error out"=w516:errorcluster)  [unwired: 5 in, 1 out]
            n186 = Send Notification(notification=w517, notifier=w513, error in (no error)=w516) -> (error out=w515:errorcluster)  [unwired: 1 out]
          }
        }
        n187 = Bundle By Name(cluster=w493, "connection ID"=w490, "data out"=w491) -> (w492:T2)
      }
      frame "Trigger" {
        # "Something Else - Replace this message with functionality for your own application."
        n188 = Unbundle By Name(w536) -> ("connection ID"=w538:refnum<k5>)
        n189 = Concatenate Strings("TRG" ("data in"), "\r") -> (w543:string)
        n190 = TCP Write(connection ID=w538, data in=w543, error in (no error)=w539) -> (connection ID out=w531:refnum<k5>, error out=w530:errorcluster)  [unwired: 1 in, 1 out]
        n191 = flat-sequence {
          tunnel: w531 -> [w551]
          tunnel: [w551] -> w528
          tunnel: w530 -> [w549]
          tunnel: [w549] -> w529
          frame #0 {
            n192 = Wait (ms)(milliseconds to wait=u32 7000) -> ()  [unwired: 1 out]
          }
        }
        n193 = TCP Read(connection ID=w528, bytes to read=256, error in (no error)=w529, 7:T8."Immediate" ("mode (standard)"), 9:5000 ("timeout ms (25000)")) -> (connection ID out=w534:refnum<k5>, data out=w533:string, error out=w537:errorcluster)
        n194 = Bundle By Name(cluster=w536, "connection ID"=w534, "data out"=w533) -> (w535:T2)
        n195 = call "Enqueue Message (Single).vi"("error in (no error)"=w537, "Message"="Trigger2", "Message Queue"=w546) -> ("error out"=w547:errorcluster)  [unwired: 7 in, 1 out]
        n196 = Merge Errors(w547) -> (w548:errorcluster)
      }
      frame "Trigger2" {
        # "Something Else - Replace this message with functionality for your own application."
        n197 = Unbundle By Name(w565) -> ("connection ID"=w566:refnum<k5>, "Camera.Prog No."=w553:string)
        n198 = Concatenate Strings("TRG" ("data in"), "\r") -> (w571:string)
        n199 = TCP Write(connection ID=w566, data in=w571, error in (no error)=w567) -> (connection ID out=w561:refnum<k5>, error out=w560:errorcluster)  [unwired: 1 in, 1 out]
        n200 = flat-sequence {
          tunnel: w561 -> [w594]
          tunnel: [w594] -> w558
          tunnel: w560 -> [w592]
          tunnel: [w592] -> w559
          frame #0 {
            n201 = Wait (ms)(milliseconds to wait=u32 7000) -> ()  [unwired: 1 out]
          }
        }
        n202 = TCP Read(connection ID=w558, bytes to read=256, error in (no error)=w559, 7:T8."Immediate" ("mode (standard)"), 9:5000 ("timeout ms (25000)")) -> (connection ID out=w563:refnum<k5>, data out=w562:string, error out=w557:errorcluster)
        "data out" <- w562
        n203 = disable-structure shown="Enabled" {
          disable-tunnel: w553 -> [_ w576]
          disable-tunnel: [w575 w576] -> w552
          frame Disabled {
            n204 = local read "Program No"() -> (w575:string)
          }
          frame Enabled {
          }
        }
        n205 = Equal?(x=w552, y="5") -> (x = y?=w554:bool)
        n206 = case shown="False" w554 {
          tunnel: w574 -> [w579 w591]
          tunnel: w557 -> [w578 w589]
          tunnel: [w577 w588] -> w556
          tunnel: w552 -> [w582 _]
          frame False {
            n207 = Equal?(x=w582, y="9") -> (x = y?=w580:bool)
            n208 = case shown="True" w580 {
              tunnel: w579 -> [_ w586]
              tunnel: w578 -> [w583 w585]
              tunnel: [w583 w584] -> w577
              frame False {
              }
              frame True {
                n209 = call-poly "Enqueue Message.vi"("error in (no error)"=w585, "Message Array"=string[] ["Update Display", "Result"], "Message Queue"=w586) -> ("error out"=w584:errorcluster)  [unwired: 7 in, 1 out]
              }
            }
          }
          frame True {
            n210 = call-poly "Enqueue Message.vi"("error in (no error)"=w589, "Message Array"=string[] ["Update Display", "SSL_Result"], "Message Queue"=w591) -> ("error out"=w588:errorcluster)  [unwired: 7 in, 1 out]
          }
        }
        n211 = Bundle By Name(cluster=w565, "connection ID"=w563, "data out"=w562) -> (w564:T2)
      }
      frame "Result" {
        n212 = Unbundle By Name(w609) -> ("data out"=w615:string, "notifier out"=w605:refnum<notifier>)
        n213 = call <userlib>:"String to 1D Array__ogtk.vi"("delimiter (Tab)"=",", "string"=w615) -> ("Array of Strings"=w614:string[])  [unwired: 9 in]
        "Array of Strings" <- w614
        n214 = Delete From Array(array=w614, index=0) -> (array with subset deleted=w599:string[])  [unwired: 1 in, 1 out]
        n215 = Array Size(array=w599) -> (size(s)=w598:i32)
        n216 = Decrement(x=w598) -> (x-1=w597:i32)
        n217 = Delete From Array(array=w599, index=w597) -> (deleted portion=→"Gray Intensity Value":string, array with subset deleted=w596:string[])  [unwired: 1 in]
        "Result Value" <- w596
        n218 = Search 1D Array(1D array=w596, element="0") -> (index of element=w612:i32)  [unwired: 1 in]
        n219 = Equal?(x=w612, y=-1) -> (x = y?=w601:bool)
        "Inspection_Result" <- w601
        n220 = Bundle By Name(cluster=T1 {"Inspection_Result 2"=FALSE, "DTU_Failed_Inspections"="DTU1_Charge_Percentage,DTU1_Vehicle_Pattern Search,DTU1_R,DTU1_Built_AI OCR,DTU1_Trip_AI OCR,DTU1_1888AI OCR,DTU1_Right_Green_Area,DTU1_Warning,DTU1_Sleep_Mode"} ("Total_Result 2"), "Inspection_Result 2"=w601, "DTU_Failed_Inspections"="") -> (w600:T1)
        n221 = case shown="False" w601 {
          tunnel: w607 -> [w620 w625]
          tunnel: [w619 w624] -> w606
          tunnel: w605 -> [_ w623]
          tunnel: w604 -> [w618 _]
          tunnel: w600 -> [_ w622]
          frame False {
            n222 = call-poly "Enqueue Message.vi"("error in (no error)"=w620, "Message"="Failed_Inspections", "Message Queue"=w618) -> ("error out"=w619:errorcluster)  [unwired: 7 in, 1 out]
          }
          frame True {
            n223 = flat-sequence {
              tunnel: w625 -> [w631]
              tunnel: w623 -> [w627]
              tunnel: w622 -> [w626]
              tunnel: [w629] -> w621
              tunnel: [w644] -> w624
              tunnel: w621 -> [w644]
              frame #0 {
                n224 = Unbundle By Name(w631) -> ("status"=w637:bool)
                n225 = call <vilib>:"Clear Errors.vi"("error in (no error)"=w631) -> ("error out"=w630:errorcluster)  [unwired: 5 in, 1 out]
                n226 = Select(t="Error" ("f"), s=w637, f="Read" ("Message")) -> (s? t:f=w633:string)
                n227 = To Variant(anything=w626) -> (Variant=w628:variant)
                n228 = Bundle(cluster=T5 {"Message"="", "Message Data"=variant} ("notification"), "Message"=w633, "Message Data"=w628) -> (w632:T5)
                n229 = Send Notification(notification=w632, notifier=w627, error in (no error)=w630) -> (error out=w629:errorcluster)  [unwired: 1 out]
              }
              frame #1 {
                n230 = Bundle(cluster=T7 {"Status"="", "Free/inuse"=FALSE, "Action"=""} ("Write"), "Status"="FREE" ("Action"), "Free/inuse"=FALSE, "Action"="IDLE" ("Status")) -> (w641:T7)
                n231 = call "FGV_camera_status.vi"("Enum"=enum16{"Init", "Read", "Write"}."Write", "Write"=w641) -> ()  [unwired: 9 in, 1 out]
              }
            }
          }
        }
        n232 = Bundle By Name(cluster=w609, "Result Value"=w596, "Total_Result"=w600) -> (w608:T2)
      }
      frame "Failed_Inspections" {
        n233 = Unbundle By Name(w652) -> ("DUT"=w647:string, "Result Value"=w669:string[], "notifier out"=w655:refnum<notifier>)
        n234 = disable-structure shown="Enabled" {
          disable-tunnel: [w690 w691] -> w668
          disable-tunnel: w647 -> [_ w691]
          frame Disabled {
            n235 = local read "Setting Value"() -> (w690:string)
          }
          frame Enabled {
          }
        }
        n236 = Decimal String To Number(string=w668) -> (number=w667:i32)  [unwired: 2 in, 1 out]
        n237 = call "Format_DTU.vi"() -> ("DTU2"=w665:string[], "DTU1"=w666:string[])  [unwired: 10 in]
        n238 = case shown="1" w667 {
          tunnel: w669 -> [_ w697 w701]
          tunnel: w666 -> [_ w696 _]
          tunnel: w665 -> [_ _ w699]
          tunnel: [_ w695 w700] -> w662
          tunnel: [_ w695 w700] -> w658
          frame 0, Default {
          }
          frame 1 {
            n239 = Build Array(w696, w697) -> (w698:string[][])
            n240 = Transpose 2D Array(2D array=w698) -> (transposed array=w695:string[][])
            "DTU1" <- w695
          }
          frame 2 {
            n241 = Build Array(w699, w701) -> (w702:string[][])
            n242 = Transpose 2D Array(2D array=w702) -> (transposed array=w700:string[][])
            "DTU 2" <- w700
          }
        }
        n243 = Index Array(array=w658, index (col)=1 ("disabled index (col)")) -> (element=w657:string[])  [unwired: 1 in]
        "Result_Values" <- w657
        n244 = call-poly <userlib>:"Search Array__ogtk.vi"("Array"=w657, "Element Data"="0") -> ("Indices of Elements"=w664:i32[])  [unwired: 7 in]
        "Fail" <- w664
        n245 = Index Array(array=w662, index (col)=0 ("disabled index (col)")) -> (element=w660:string[])  [unwired: 1 in]
        "Inspection_names" <- w660
        n246 = for {
          tunnel: w660 -> [w694]
          tunnel: w664 -> [w693] mode=indexing
          tunnel: [w692] -> w654 mode=indexing
          n247 = Index Array(array=w694, index=w693) -> (element=w692:string)
        }
        "DTU_Failed_Inspections_Array" <- w654
        n248 = Unbundle By Name(w652) -> ("Inspection_Result"=w651:bool)
        n249 = call <userlib>:"1D Array to String__ogtk.vi"("delimiter (Tab)"=",", "Array of Strings"=w654) -> ("delimited string"=w650:string)  [unwired: 9 in]
        "DTU_Failed_Inspections" <- w650
        n250 = Bundle By Name(cluster="Total_Result", "Inspection_Result 2"=w651, "DTU_Failed_Inspections"=w650) -> (w649:T1)
        n251 = flat-sequence {
          tunnel: w655 -> [w674]
          tunnel: w645 -> [w673]
          tunnel: w649 -> [w671]
          tunnel: [w672] -> w646
          tunnel: w645 -> [w670]
          tunnel: [w689] -> w653
          tunnel: w646 -> [w689]
          frame #0 {
            n252 = Unbundle By Name(w673) -> ("status"=w682:bool)
            n253 = To Variant(anything=w671) -> (Variant=w675:variant)
            n254 = Select(t="Error" ("f"), s=w682, f="Read" ("Message")) -> (s? t:f=w678:string)
            n255 = Bundle By Name(cluster=T5 {"Message"="", "Message Data"=variant} ("notification"), "Message"=w678, "Message Data"=w675) -> (w677:T5)
            n256 = call <vilib>:"Clear Errors.vi"("error in (no error)"=w670) -> ("error out"=w676:errorcluster)  [unwired: 5 in, 1 out]
            n257 = Send Notification(notification=w677, notifier=w674, error in (no error)=w676) -> (error out=w672:errorcluster)  [unwired: 1 out]
          }
          frame #1 {
            n258 = Bundle(cluster=T7 {"Status"="", "Free/inuse"=FALSE, "Action"=""} ("Write"), "Status"="FREE" ("Action"), "Free/inuse"=FALSE, "Action"="IDLE" ("Status")) -> (w686:T7)
            n259 = call "FGV_camera_status.vi"("Enum"=enum16{"Init", "Read", "Write"}."Write", "Write"=w686) -> ()  [unwired: 9 in, 1 out]
          }
        }
      }
      frame "SSL_Result" {
        n260 = Unbundle By Name(w715) -> ("data out"=w708:string, "notifier out"=w713:refnum<notifier>)  [unwired: 1 out]
        "RX,RY" <- w708
        n261 = Spreadsheet String To Array(delimiter (Tab)=",", format string="%s", spreadsheet string=w708, array type (2D Dbl)=string[] []) -> (array=w706:string[])
        n262 = Search 1D Array(1D array=w706, element="1") -> (index of element=w704:i32)  [unwired: 1 in]
        n263 = case shown="1" w704 {
          tunnel: ["RX" "RY"] -> w703
          frame 0, Default {
          }
          frame 1 {
          }
        }
        "RX/RY" <- w703
        n264 = flat-sequence {
          tunnel: w713 -> [w722]
          tunnel: w712 -> [w721]
          tunnel: [w720] -> w714
          tunnel: w712 -> [w719]
          tunnel: w703 -> [w718]
          tunnel: [w737] -> w711
          tunnel: w714 -> [w737]
          frame #0 {
            n265 = Unbundle By Name(w721) -> ("status"=w730:bool)
            n266 = To Variant(anything=w718) -> (Variant=w723:variant)
            n267 = Select(t="Error" ("f"), s=w730, f="Read" ("Message")) -> (s? t:f=w726:string)
            n268 = Bundle By Name(cluster=T5 {"Message"="", "Message Data"=variant} ("notification"), "Message"=w726, "Message Data"=w723) -> (w725:T5)
            n269 = call <vilib>:"Clear Errors.vi"("error in (no error)"=w719) -> ("error out"=w724:errorcluster)  [unwired: 5 in, 1 out]
            n270 = Send Notification(notification=w725, notifier=w722, error in (no error)=w724) -> (error out=w720:errorcluster)  [unwired: 1 out]
          }
          frame #1 {
            n271 = Bundle(cluster=T7 {"Status"="", "Free/inuse"=FALSE, "Action"=""} ("Write"), "Status"="FREE" ("Action"), "Free/inuse"=FALSE, "Action"="IDLE" ("Status")) -> (w734:T7)
            n272 = call "FGV_camera_status.vi"("Enum"=enum16{"Init", "Read", "Write"}."Write", "Write"=w734) -> ()  [unwired: 9 in, 1 out]
          }
        }
      }
      frame "Update Display" {
        # "Update Display - Convert the message data to a string to display in the Data Display indicator."
        n273 = Unbundle By Name(w739) -> ("data out"=→"Display <Replace Me>":string)
        n274 = Merge Errors(w740) -> (w741:errorcluster)
      }
      frame "Error" {
        # "#CodeRecommended - If you ever change the name of this \"Error\" message, you'll need to update the name in the Check Loop Error.vi as well."
        # "#CodeRecommended - Consider creating a system for logging errors in some way. These errors are for notification purposes only. Handling of specific errors should be performed in the message frames that generated the error."
        # "Error - Display an error dialog. This message is sent by the \"Error Handler\" VIs at the end of other loops in this application."
        n275 = Variant To Data(error in=w750, type=errorcluster {"status"=FALSE, "code"=0, "source"=""} ("error constant"), Variant=w748) -> (data=w746:errorcluster, error out=w745:errorcluster)
        n276 = call <vilib>:"Simple Error Handler.vi"("error in (no error)"=w746) -> ()  [unwired: 4 in, 5 out]
        n277 = call "FGV_camera_status.vi"("Enum"=enum16{"Init", "Read", "Write"}."Write", "Write"=T7 {"Status"="Error", "Free/inuse"=FALSE, "Action"=""}) -> ()  [unwired: 9 in, 1 out]
        n278 = Merge Errors(w745) -> (w744:errorcluster)
      }
      frame "Reset" {
        # "Reset"
        n279 = call "FGV_camera_status.vi"("Enum"=enum16{"Init", "Read", "Write"}."Write", "Write"=T7 {"Status"="", "Free/inuse"=FALSE, "Action"=""}) -> ()  [unwired: 9 in, 1 out]
        n280 = Merge Errors(w755) -> (w753:errorcluster)
      }
      frame "Confirm Quit" {
        # "Confirm Quit - Message that can confirm whether or not the user wants to exit the application."
        n281 = Unbundle By Name(w756) -> ("notifier out"=w760:refnum<notifier>)
        n282 = Release Notifier(notifier=w760, force destroy? (F)=TRUE, error in (no error)=w758) -> (error out=w757:errorcluster)  [unwired: 2 out]
        n283 = call "Enqueue Message (Single).vi"("Priority Message? (F)"=TRUE, "error in (no error)"=w757, "Message"="Exit", "Message Queue"=w763) -> ("error out"=w764:errorcluster)  [unwired: 6 in, 1 out]
      }
      frame "Exit" {
        # "Stop the VI"
        # "Release the message queue reference"
        # "Exit - Exit the application."
        n284 = Variant To Data(type=errorcluster {"status"=FALSE, "code"=0, "source"=""} ("error constant"), Variant=w772) -> (data=w773:errorcluster)  [unwired: 1 in, 1 out]
        n285 = call <vilib>:"Simple Error Handler.vi"("error in (no error)"=w773) -> ()  [unwired: 4 in, 5 out]
        n286 = Unbundle By Name(w770) -> ("connection ID"=w769:refnum<k5>)
        n287 = TCP Close Connection(connection ID=w769, error in (no error)=w771) -> (error out=w768:errorcluster)  [unwired: 1 in, 1 out]
        n288 = call "Fire User Event - Stop.vi"("User Event - Stop"=w775) -> ("error out"=w766:errorcluster)  [unwired: 10 in]
        n289 = call <vilib>:"Clear Errors.vi"("error in (no error)"=w768) -> ("error out"=w767:errorcluster)  [unwired: 5 in, 1 out]
        n290 = call <vilib>:"Clear Errors.vi"("error in (no error)"=w766) -> ("error out"=w765:errorcluster)  [unwired: 5 in, 1 out]
        n291 = Release Queue(queue=w779, error in (no error)=w767) -> (error out=w777:errorcluster)  [unwired: 1 in, 2 out]
        n292 = Merge Errors(w765, w777) -> (w776:errorcluster)
      }
      frame Default {
        # "'Default' case only runs if there is a message that isn't defined in any of the other cases.  Output a programming error."
        n293 = xnode "Error Ring"("parameter 0"=w780) -> ("error out"=w781:errorcluster)
      }
    }
    n294 = call "Error Handler - Message Handling Loop.vi"("error in (no error)"=w24, "Message Queue"=w26) -> ("dup error in"=w25:errorcluster)  [unwired: 8 in, 1 out]
  }
  n295 = while {
    tunnel: w5 -> [w796]
    shift-right: [w794] -> w18
    shift-left: w15 -> [w795]
    tunnel: [w790] -> w16
    stop <- w792 stop-if-true
    # "Event Handling Loop"
    n296 = event shown="[4] \"Trigger\": Value Change" {
      selector: w795 -> [_ _ _ _ _ _]
      dyn-events: [_ _ _ _ _ _] -> w794
      timeout: _ -> [_ _ _ _ _ _]
      tunnel: [_ _ _ TRUE ("Discard?") _ _] -> w792
      tunnel: w796 -> [w801 w803 w808 w811 w815 w819]
      tunnel: [w800 _ w807 _ w812 w818] -> w793
      tunnel: [w799 w803 w806 w811 w814 w817] -> w791
      event Panel Close? {
        # "Send the 'Confirm Quit' message if the user closes the panel of the VI. Discard the event so the 'Confirm Quit' message has a chance to run."
        n297 = event-data() -> ()  [unwired: 1 in, 1 out]
        n298 = call "Enqueue Message (Single).vi"("Priority Message? (F)"=TRUE, "Message"="Confirm Quit", "Message Queue"=w801) -> ("error out"=w800:errorcluster, "dup Message Queue"=w799:refnum<queue>)  [unwired: 7 in]
        n299 = event-data("Discard?"=TRUE) -> ()  [unwired: 1 in, 1 out]
      }
      event Application Instance Close {
        # "#CodeRecommended - When a project closes, all VIs within that project are aborted and leave memory. However, any code placed in this event frame is guaranteed to run to completion, so add any cleanup code that absolutely must happen here."
        n300 = event-data() -> ()  [unwired: 1 in, 1 out]
      }
      event "Exit": Value Change {
        n301 = event-data() -> ()  [unwired: 1 in, 1 out]
        n302 = call "Enqueue Message (Single).vi"("Priority Message? (F)"=TRUE, "Message"="Exit", "Message Queue"=w808) -> ("error out"=w807:errorcluster, "dup Message Queue"=w806:refnum<queue>)  [unwired: 7 in]
      }
      event User Event {
        # "The Message Handling Loop processed an \"Exit\" message, which fired this event to stop the Event Handling Loop."
        n303 = event-data() -> ()  [unwired: 1 in, 1 out]
        n304 = local write "Display <Replace Me>"("\"Exit\" button pressed" ("VI Stopped")) -> ()
      }
      event "Trigger": Value Change {
        n305 = event-data() -> ()  [unwired: 1 in, 1 out]
        n306 = call "Enqueue Message (Single).vi"("Message"="Trigger", "Message Queue"=w815) -> ("error out"=w812:errorcluster, "dup Message Queue"=w814:refnum<queue>)  [unwired: 8 in]
      }
      event "Change_Program": Value Change {
        n307 = event-data() -> ()  [unwired: 1 in, 1 out]
        n308 = call "Enqueue Message (Single).vi"("Message"="Change_Program", "Message Queue"=w819) -> ("error out"=w818:errorcluster, "dup Message Queue"=w817:refnum<queue>)  [unwired: 8 in]
      }
    }
    n309 = call "Error Handler - Event Handling Loop.vi"("error in (no error)"=w793, "Message Queue"=w791) -> ("dup error in"=w790:errorcluster)  [unwired: 8 in, 1 out]
  }
  n310 = Unregister For Events(event registration refnum=w18, error in=w16) -> (error out=w19:errorcluster)
  n311 = Merge Errors(w19, w22) -> (w20:errorcluster)
  n312 = call "Destroy User Event - Stop.vi"("error in (no error)"=w20, "User Event - Stop"=w14) -> ("error out"=w17:errorcluster)  [unwired: 9 in]
  n313 = disable-structure shown="Default" {
    disable-tunnel: w17 -> [_ _]
    frame condition #0 (active) {
    }
    frame condition #1 {
      # "Call Quit LabVIEW if running as a built application."
      n314 = Quit LabVIEW() -> ()  [unwired: 1 in]
    }
  }
